vi "tio32_Read_ADS1100.vi"(0 "VISA resource name":refnum<visa-resource-name>, 5 "Board address":i32=4660 format="%x", 7 "ADS number":i32=1, 9 "mode":i32=1, 11 "error in (no error)":errorcluster, 12 "User Ref":dbl=1.0) -> (4 "VISA resource name out":refnum<visa-resource-name>, 6 "return":i32=666, 8 "code":i32=666, 10 "value":dbl=666.0, 15 "error out":errorcluster)   [LabVIEW 2011]
uses:
  l_pse_dll/Tio32.dll
panel:
  # "tio32_Read_ADS1100"
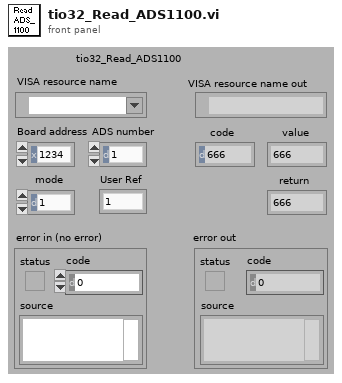
[diagram p1: front panel]
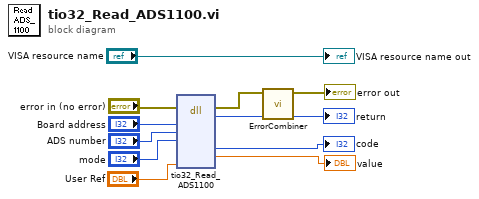
[diagram p0: block diagram]
diagram:
  n1 = dll-call lib="C:/Users/Ikaika's/Documents/DCC/Apps/INA231/INA231-SFT-rev1/INA231-Sourcecode-rev1/INA231/Shell Resources/l_pse_dll/Tio32.dll" fn="tio32_Read_ADS1100" label="tio32_Read_ADS1100()"(error in="error in (no error)", "adr"="Board address", "adsNo"="ADS number", "mode"="mode", "refUser"="User Ref") -> (error out=w7:errorcluster, "Rückgabetyp"=w8:i32, "pCode"=→"code":i32, "pVal"=→"value":dbl)  [unwired: 8 in, 1 out]
  n2 = call "ErrorCombiner.vi"("Return In"=w8, "error in (no error)"=w7) -> ("Return Out"=→"return":i32, "error out"=→"error out":errorcluster)  [unwired: 8 in]
  "VISA resource name out" <- "VISA resource name"
